vi "Práctica10_USB.vi"() -> ()   [LabVIEW 2018]
panel:
  out "VISA resource name out":refnum<visa-resource-name>
  out "error out 2":errorcluster
  in  "error in (no error) 2":errorcluster
  in  "length (0)":u16
  in  "request":i16
  in  "VISA resource name":refnum<visa-resource-name>
  out "error out":errorcluster
  out "VISA USB Intr Event out":refnum<visa-resource-name>
  in  "error in (no error)":errorcluster
  in  "VISA USB Intr Event":refnum<visa-resource-name>
  # "Anahí Montserrat Vázquez Padilla\nComunicación por USB\n30/04/2024"
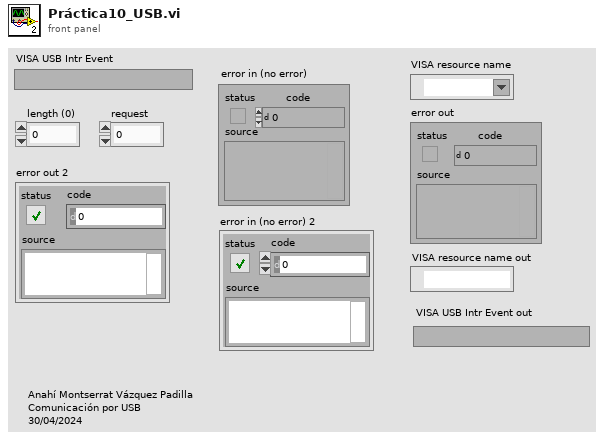
[diagram p1: front panel]
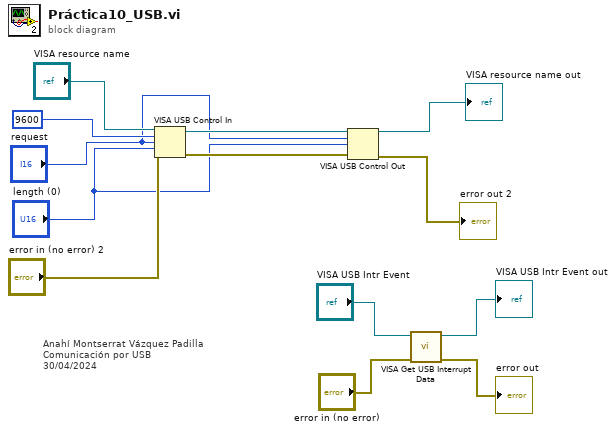
[diagram p0: block diagram]
diagram:
  # "Anahí Montserrat Vázquez Padilla\nComunicación por USB\n30/04/2024"
  n1 = VISA USB Control In(0:"VISA resource name", 5:i16 9600 ("request type"), 7:"request", 9:"length (0)", 11:"error in (no error) 2") -> (4:w3:refnum<visa-resource-name>, 15:w6:errorcluster)  [unwired: 2 in, 1 out]
  n2 = VISA USB Control Out(0:w3, 5:"request", 7:"length (0)", 11:w6) -> (4:→"VISA resource name out":refnum<visa-resource-name>, 15:→"error out 2":errorcluster)  [unwired: 3 in]
  n3 = call <vilib>:"VISA Get USB Interrupt Data.vi"("error in (no error)"="error in (no error)", "VISA USB Intr Event"="VISA USB Intr Event") -> ("error out"=→"error out":errorcluster, "VISA USB Intr Event out"=→"VISA USB Intr Event out":refnum<visa-resource-name>)  [unwired: 7 in, 1 out]
